vi "WT1800.vi"(7 "simulazione":bool, 8 "error in (no error)":errorcluster, 11 "Queue Name":string="WT1800_Q") -> (0 "error out":errorcluster, 2 "Stopped":bool)   [LabVIEW 2019]
uses:
  TypeDef/MISURE WT.ctl
  TypeDef/DEVICE NAME.ctl
  <vilib>/Utility/file.llb/Read From Spreadsheet File (string).vi
  <instrlib>/Yokogawa WT1800 Series/Public/Data/Low Level/Fetch Measurement (Normal).vi
  Globals.vi
  <instrlib>/Yokogawa WT1800 Series/Yokogawa WT1800 Series.lvlib
panel:
  out "Measurement":dbl[](array[numeric])
  in  "Number of Item (15)":i32=90 min=1 max=255
  in  "WT1800 Config ing":T1={"Wiring A (0: 1P2W)"=0, "Wiring B (0: 1P2W)"=0, "Wiring C (0: 1P2W)"=0, "V Range (12: 1000)"=12, "V Element (0: All)"=0, "A Element (0: All)"=0, "A Range (9: 5A)"=9, "A Sensor Ratio(mV/A) (10.0000) "=10.0, "Zero Cross Filter (0: OFF)"=0, "Line Filter (0: OFF)"=0, "PT Ratio (1.0000)"=1.0, "Scaling (F: OFF)"=FALSE, "CT Ratio (1.0000)"=1.0, "Scaling Factor (1.0000)"=1.0, "Filter Element (0: All)"=0, "Display Format (0: Numeric)"=0, "Normal Item Amount (1: 4)"=1, "Harmonics Item Amount (1: 4)"=1, "Average Type (0: OFF)"=0, "Average Count (2: 8)"=2, "A Range (9: 5A) 2"=9, "A Sensor Ratio(mV/A) (10.0000)  2"=10.0, "Zero Cross Filter (0: OFF) 2"=0, "Line Filter (0: OFF) 2"=0, "PT Ratio (1.0000) 2"=1.0, "Scaling (F: OFF) 2"=FALSE, "CT Ratio (1.0000) 2"=1.0, "Scaling Factor (1.0000) 2"=1.0, "CUT OFF FREQ"=0.0} {"Scaling Factor (1.0000) 2" min=0.0001 max=99999.9999 step=0.0001 format="%.4f"; "CT Ratio (1.0000) 2" min=0.0001 max=99999.9999 step=0.0001 format="%.4f"; "PT Ratio (1.0000) 2" min=0.0001 max=99999.9999 step=0.0001 format="%.4f"; "Line Filter (0: OFF) 2" items=["OFF", "500Hz", "5.5kHz"]; "Zero Cross Filter (0: OFF) 2" items=["OFF", "500Hz"]; "A Sensor Ratio(mV/A) (10.0000)  2" min=0.0001 max=99999.9999 step=0.0001 format="%.4f"; "A Range (9: 5A) 2" items=["AUTO", "10 mA", "20 mA", "50 mA", "100 mA", "200 mA", "500 mA", "1 A", "2 A", "5 A", "10 A", "20 A", "50 A", "S-AUTO", "50 mV", "100 mV", "250 mV", "500 mV", "1 V", "2.5 V", "5 V", "10 V"]; "Average Count (2: 8)" items=["2", "4", "8", "16", "32", "64", "128", "256"]; "Average Type (0: OFF)" items=["OFF", "Linear", "Exponent"]; "Harmonics Item Amount (1: 4)" items=["-", "4", "8", "16", "Single List", "Dual List", "Sigma List"]; "Normal Item Amount (1: 4)" items=["ALL", "4", "8", "16", "42", "78"]; "Display Format (0: Numeric)" items=["Numeric", "Wave", "Bar", "Vector", "Trend", "Numeric & Wave", "Numeric & Bar", "Numeric & Trend", "Wave & Bar", "Wave & Trend", "Bar & Trend", "Information"]; "Filter Element (0: All)" items=["All", "Element 1", "Element 2", "Element 3", "Element 4", "Element 5", "Element 6"]; "Scaling Factor (1.0000)" min=0.0001 max=99999.9999 step=0.0001 format="%.4f"; "CT Ratio (1.0000)" min=0.0001 max=99999.9999 step=0.0001 format="%.4f"; "PT Ratio (1.0000)" min=0.0001 max=99999.9999 step=0.0001 format="%.4f"; "Line Filter (0: OFF)" items=["OFF", "500Hz", "5.5kHz"]; "Zero Cross Filter (0: OFF)" items=["OFF", "500Hz"]; "A Sensor Ratio(mV/A) (10.0000)" min=0.0001 max=99999.9999 step=0.0001 format="%.4f"; "A Range (9: 5A)" items=["AUTO", "10 mA", "20 mA", "50 mA", "100 mA", "200 mA", "500 mA", "1 A", "2 A", "5 A", "10 A", "20 A", "50 A", "S-AUTO", "50 mV", "100 mV", "250 mV", "500 mV", "1 V", "2.5 V", "5 V", "10 V"]; "A Element (0: All)" items=["All", "Element 1", "Element 2", "Element 3", "Element 4", "Element 5", "Element 6"]; "V Element (0: All)" items=["All", "Element 1", "Element 2", "Element 3", "Element 4", "Element 5", "Element 6"]; "V Range (12: 1000)" items=["AUTO", "1.5", "3", "6", "10", "15", "30", "60", "100", "150", "300", "600", "1000"]; "Wiring C (0: 1P2W)" items=["1P2W", "1P3W", "3P3W", "3P4W", "3V3A", "NONE"]; "Wiring B (0: 1P2W)" items=["1P2W", "1P3W", "3P3W", "3P4W", "3V3A", "NONE"]; "Wiring A (0: 1P2W)" items=["1P2W", "1P3W", "3P3W", "3P4W", "3V3A"]}
  out "MISURE WT":T2
  out "VISA resource name":refnum<visa-resource-name>
  out "STATO":string
  out "LOOP TIME (ms)":u32
  # "ON\nOFF"
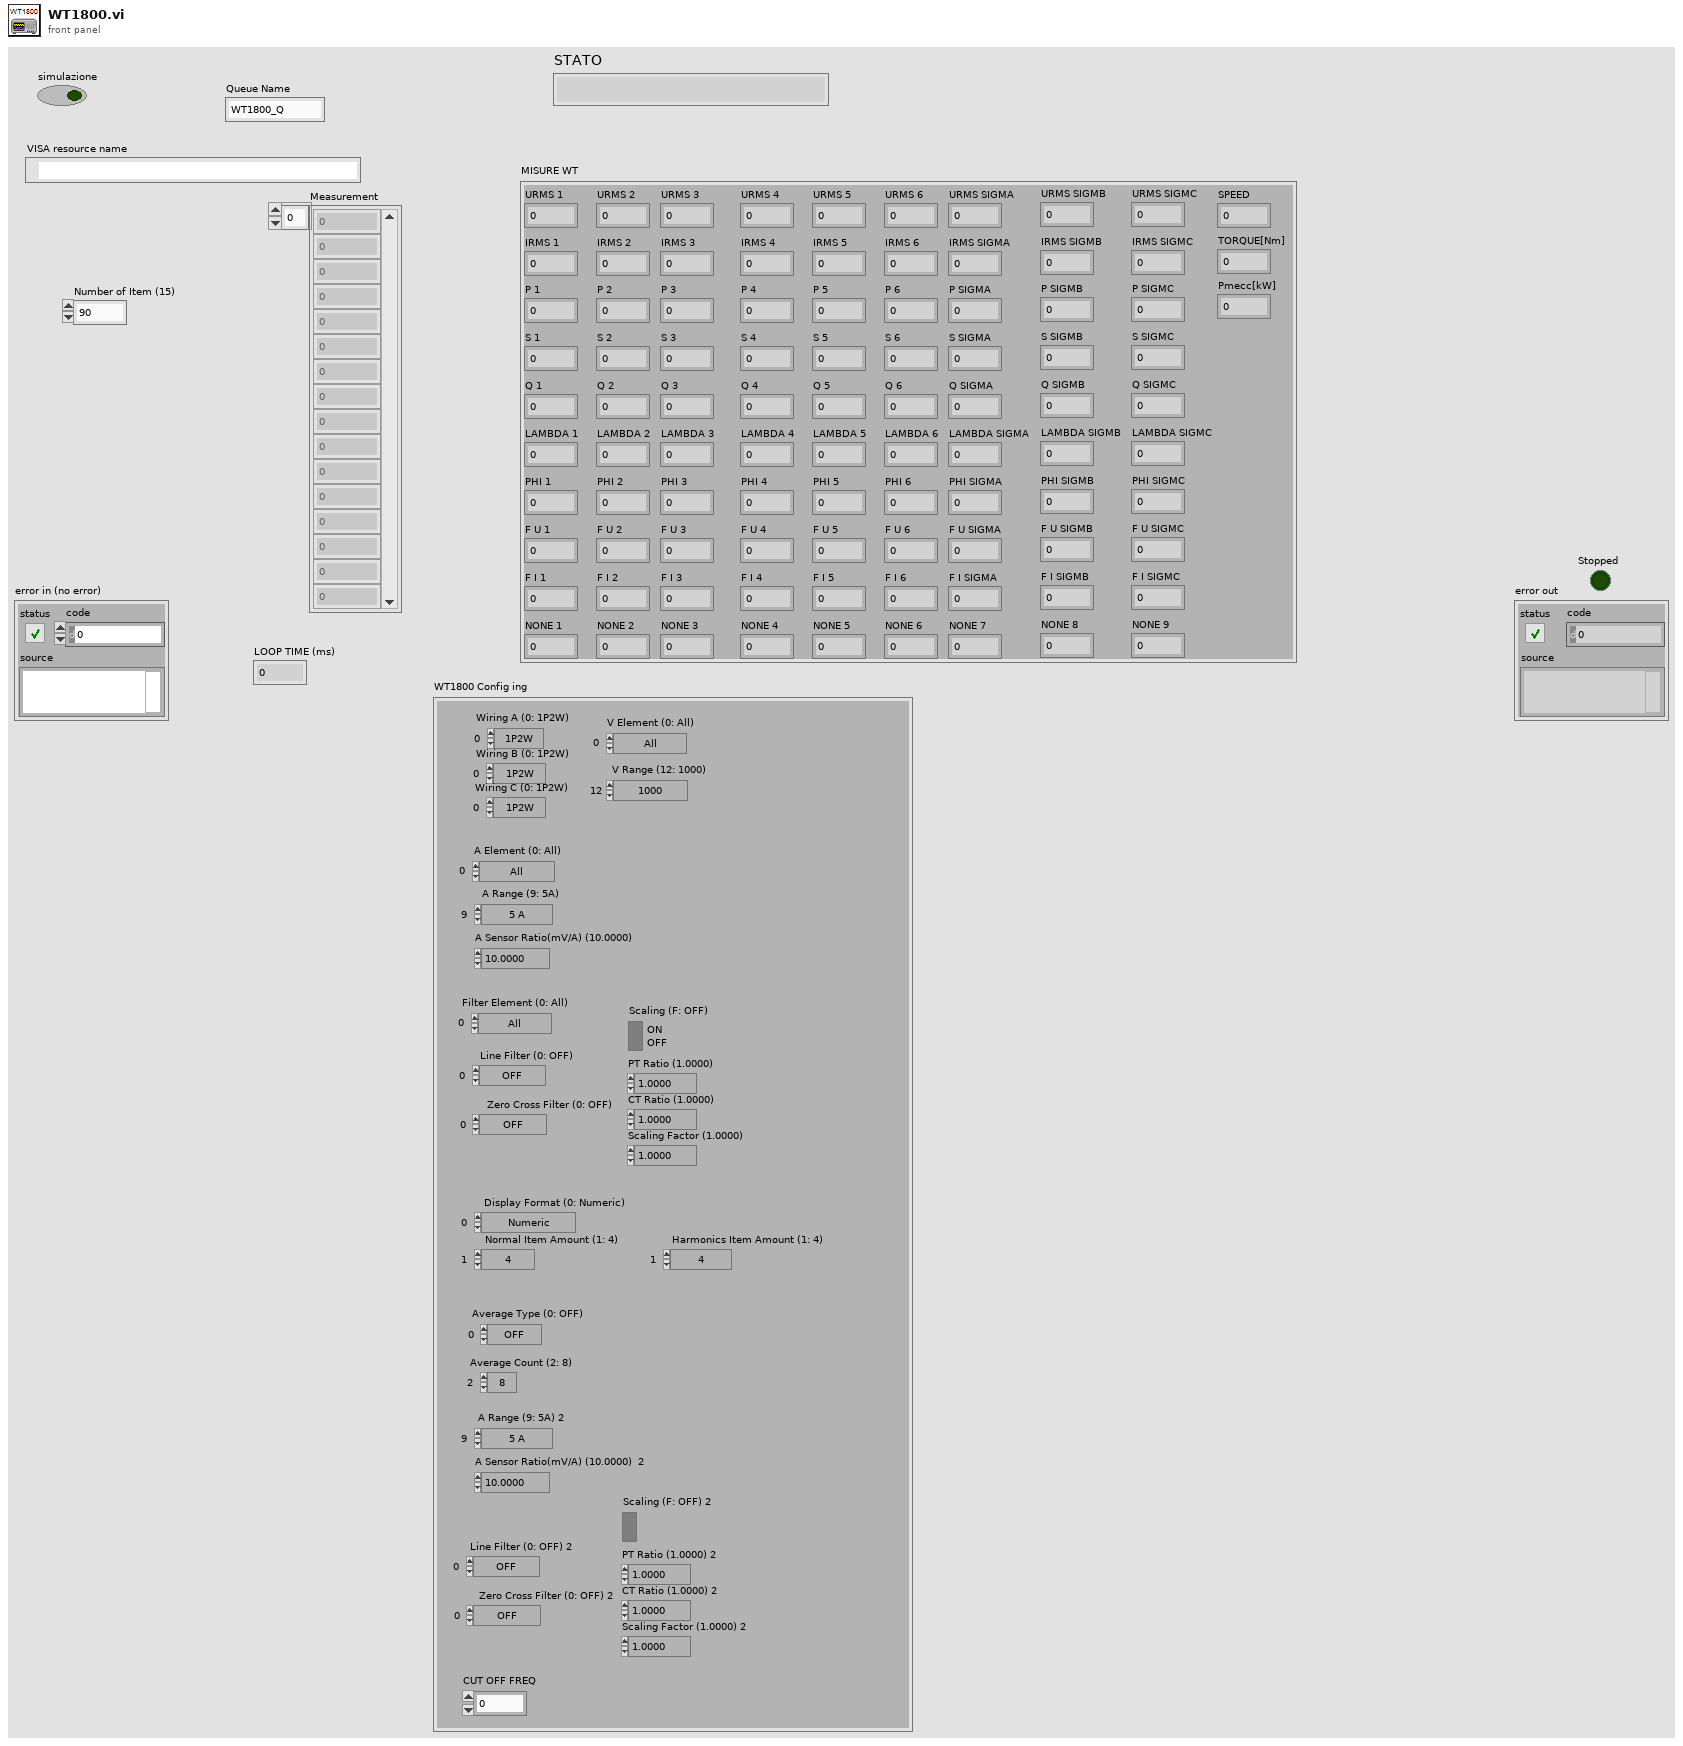
[diagram p1: front panel]
types:
  T1 = cluster{"Wiring A (0: 1P2W)":u16, "Wiring B (0: 1P2W)":u16, "Wiring C (0: 1P2W)":u16, "V Range (12: 1000)":u16, "V Element (0: All)":u16, "A Element (0: All)":u16, "A Range (9: 5A)":u16, "A Sensor Ratio(mV/A) (10.0000) ":dbl, "Zero Cross Filter (0: OFF)":u16, "Line Filter (0: OFF)":u16, "PT Ratio (1.0000)":dbl, "Scaling (F: OFF)":bool, "CT Ratio (1.0000)":dbl, "Scaling Factor (1.0000)":dbl, "Filter Element (0: All)":u16, "Display Format (0: Numeric)":u16, "Normal Item Amount (1: 4)":u16, "Harmonics Item Amount (1: 4)":u16, "Average Type (0: OFF)":u16, "Average Count (2: 8)":u16, "A Range (9: 5A) 2":u16, "A Sensor Ratio(mV/A) (10.0000)  2":dbl, "Zero Cross Filter (0: OFF) 2":u16, "Line Filter (0: OFF) 2":u16, "PT Ratio (1.0000) 2":dbl, "Scaling (F: OFF) 2":bool, "CT Ratio (1.0000) 2":dbl, "Scaling Factor (1.0000) 2":dbl, "CUT OFF FREQ":dbl}
  T2 = typedef "MISURE WT.ctl" = cluster{"URMS 1":dbl, "IRMS 1":dbl, "P 1":dbl, "S 1":dbl, "Q 1":dbl, "LAMBDA 1":dbl, "PHI 1":dbl, "F U 1":dbl, "F I 1":dbl, "NONE 1":dbl, "URMS 2":dbl, "IRMS 2":dbl, "P 2":dbl, "S 2":dbl, "Q 2":dbl, "LAMBDA 2":dbl, "PHI 2":dbl, "F U 2":dbl, "F I 2":dbl, "NONE 2":dbl, "URMS 3":dbl, "IRMS 3":dbl, "P 3":dbl, "S 3":dbl, "Q 3":dbl, "LAMBDA 3":dbl, "PHI 3":dbl, "F U 3":dbl, "F I 3":dbl, "NONE 3":dbl, "URMS 4":dbl, "IRMS 4":dbl, "P 4":dbl, "S 4":dbl, "Q 4":dbl, "LAMBDA 4":dbl, "PHI 4":dbl, "F U 4":dbl, "F I 4":dbl, "NONE 4":dbl, "URMS 5":dbl, "IRMS 5":dbl, "P 5":dbl, "S 5":dbl, "Q 5":dbl, "LAMBDA 5":dbl, "PHI 5":dbl, "F U 5":dbl, "F I 5":dbl, "NONE 5":dbl, "URMS 6":dbl, "IRMS 6":dbl, "P 6":dbl, "S 6":dbl, "Q 6":dbl, "LAMBDA 6":dbl, "PHI 6":dbl, "F U 6":dbl, "F I 6":dbl, "NONE 6":dbl, "URMS SIGMA":dbl, "IRMS SIGMA":dbl, "P SIGMA":dbl, "S SIGMA":dbl, "Q SIGMA":dbl, "LAMBDA SIGMA":dbl, "PHI SIGMA":dbl, "F U SIGMA":dbl, "F I SIGMA":dbl, "NONE 7":dbl, "URMS SIGMB":dbl, "IRMS SIGMB":dbl, "P SIGMB":dbl, "S SIGMB":dbl, "Q SIGMB":dbl, "LAMBDA SIGMB":dbl, "PHI SIGMB":dbl, "F U SIGMB":dbl, "F I SIGMB":dbl, "NONE 8":dbl, "URMS SIGMC":dbl, "IRMS SIGMC":dbl, "P SIGMC":dbl, "S SIGMC":dbl, "Q SIGMC":dbl, "LAMBDA SIGMC":dbl, "PHI SIGMC":dbl, "F U SIGMC":dbl, "F I SIGMC":dbl, "NONE 9":dbl, "SPEED":dbl, "TORQUE[Nm]":dbl, "Pmecc[kW]":dbl}
  T3 = typedef "DEVICE NAME.ctl" = enum16{"WATTMETRO", "APLUS", "PLC BANCO 1", "PLC RACK", "PLC BANCO 2", "PS", "NI cDAQ", "RESISTOMAT"}
  T4 = cluster{"Array of elements":cluster{"String":string, "variant":variant}[], "Single element":cluster{"String":string, "variant":variant}, "enque at\nopposite end (F)":bool, "no replications (F)":bool}
  T5 = cluster{"Measurement[0]":dbl, "Measurement[1]":dbl, "Measurement[2]":dbl, "Measurement[3]":dbl, "Measurement[4]":dbl, "Measurement[5]":dbl, "Measurement[6]":dbl, "Measurement[7]":dbl, "Measurement[8]":dbl, "Measurement[9]":dbl, "Measurement[10]":dbl, "Measurement[11]":dbl, "Measurement[12]":dbl, "Measurement[13]":dbl, "Measurement[14]":dbl, "Measurement[15]":dbl, "Measurement[16]":dbl, "Measurement[17]":dbl, "Measurement[18]":dbl, "Measurement[19]":dbl, "Measurement[20]":dbl, "Measurement[21]":dbl, "Measurement[22]":dbl, "Measurement[23]":dbl, "Measurement[24]":dbl, "Measurement[25]":dbl, "Measurement[26]":dbl, "Measurement[27]":dbl, "Measurement[28]":dbl, "Measurement[29]":dbl, "Measurement[30]":dbl, "Measurement[31]":dbl, "Measurement[32]":dbl, "Measurement[33]":dbl, "Measurement[34]":dbl, "Measurement[35]":dbl, "Measurement[36]":dbl, "Measurement[37]":dbl, "Measurement[38]":dbl, "Measurement[39]":dbl, "Measurement[40]":dbl, "Measurement[41]":dbl, "Measurement[42]":dbl, "Measurement[43]":dbl, "Measurement[44]":dbl, "Measurement[45]":dbl, "Measurement[46]":dbl, "Measurement[47]":dbl, "Measurement[48]":dbl, "Measurement[49]":dbl, "Measurement[50]":dbl, "Measurement[51]":dbl, "Measurement[52]":dbl, "Measurement[53]":dbl, "Measurement[54]":dbl, "Measurement[55]":dbl, "Measurement[56]":dbl, "Measurement[57]":dbl, "Measurement[58]":dbl, "Measurement[59]":dbl, "Measurement[60]":dbl, "Measurement[61]":dbl, "Measurement[62]":dbl, "Measurement[63]":dbl, "Measurement[64]":dbl, "Measurement[65]":dbl, "Measurement[66]":dbl, "Measurement[67]":dbl, "Measurement[68]":dbl, "Measurement[69]":dbl, "Measurement[70]":dbl, "Measurement[71]":dbl, "Measurement[72]":dbl, "Measurement[73]":dbl, "Measurement[74]":dbl, "Measurement[75]":dbl, "Measurement[76]":dbl, "Measurement[77]":dbl, "Measurement[78]":dbl, "Measurement[79]":dbl, "Measurement[80]":dbl, "Measurement[81]":dbl, "Measurement[82]":dbl, "Measurement[83]":dbl, "Measurement[84]":dbl, "Measurement[85]":dbl, "Measurement[86]":dbl, "Measurement[87]":dbl, "Measurement[88]":dbl, "Measurement[89]":dbl, "Measurement[90]":dbl, "Measurement[91]":dbl, "Measurement[92]":dbl}
  T6 = enum32{"Invalid", "Standard", "Closed", "Hidden", "Minimized", "Maximized"}
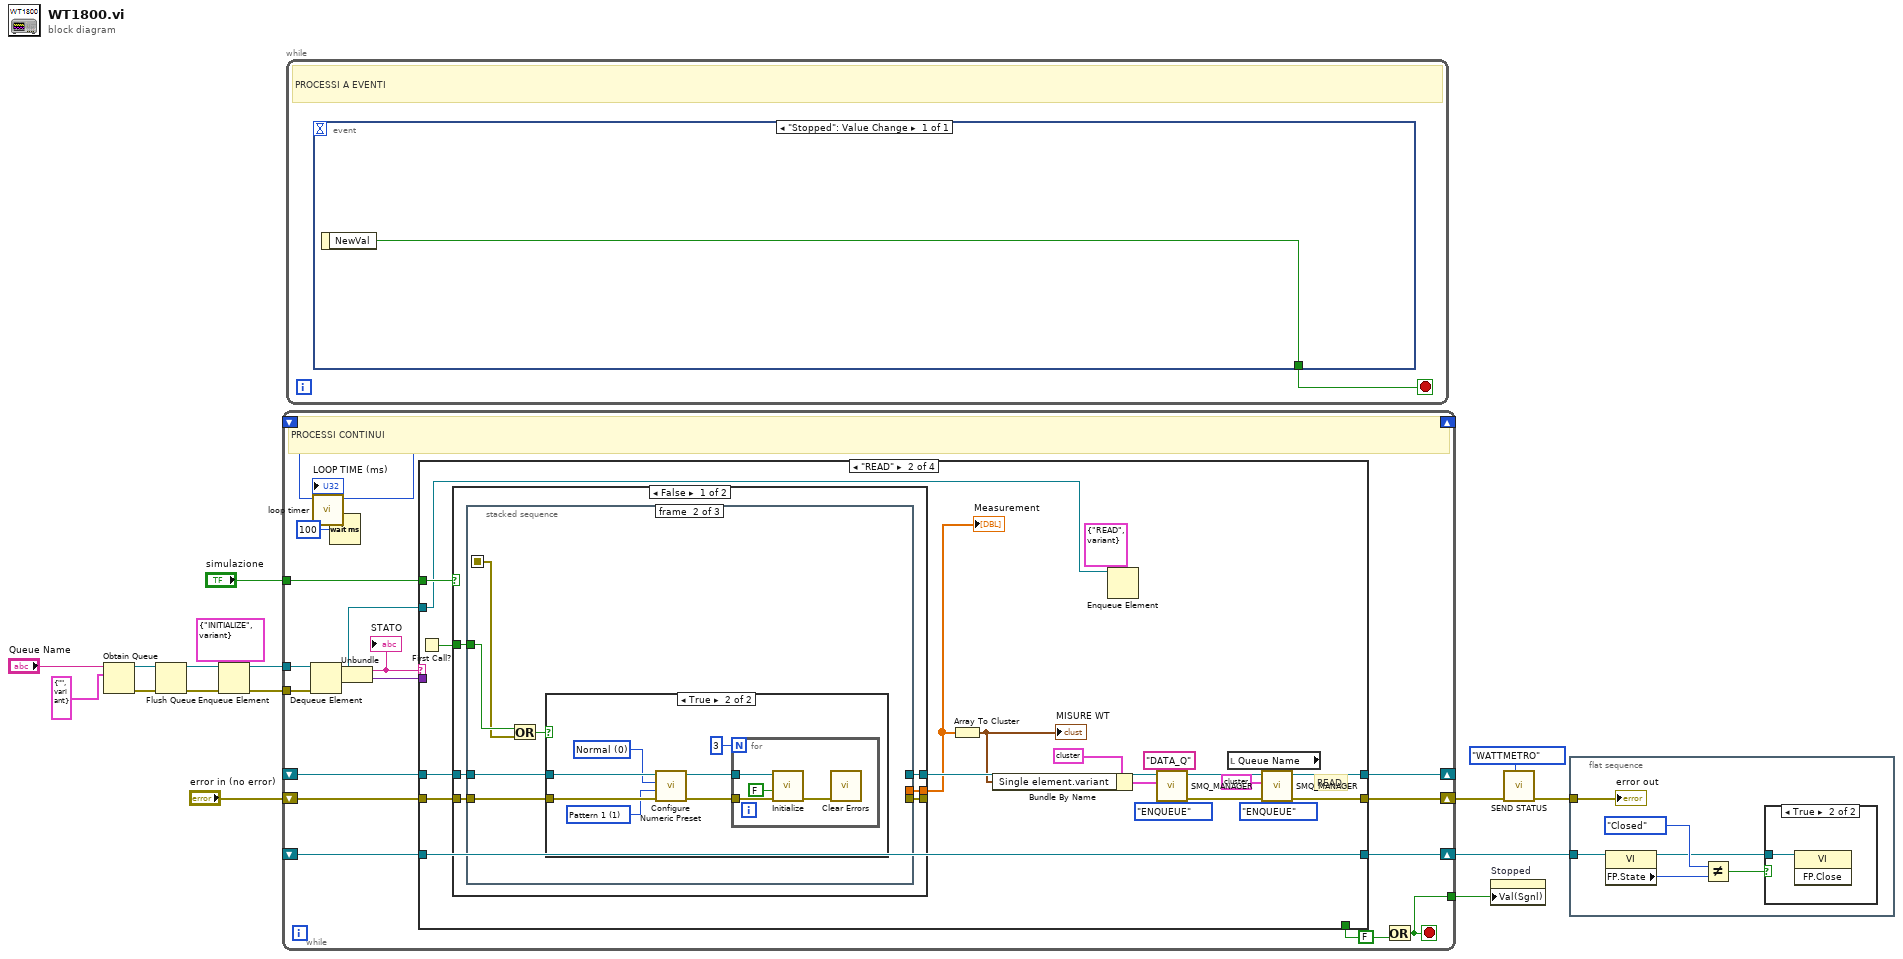
[diagram p0: block diagram]
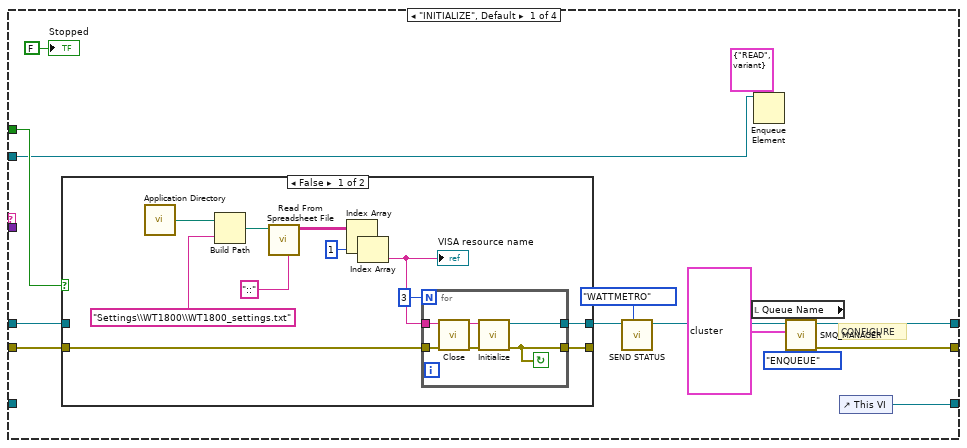
[diagram p3: hidden frame]
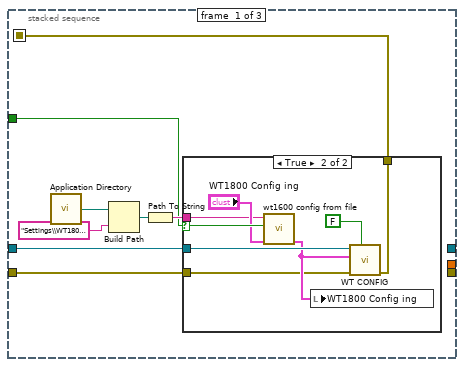
[diagram p5: hidden frame]
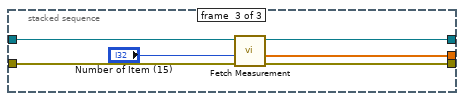
[diagram p8: hidden frame]
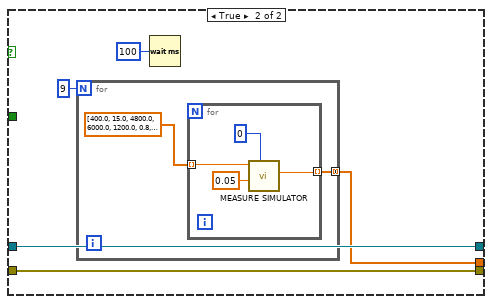
[diagram p9: hidden frame]
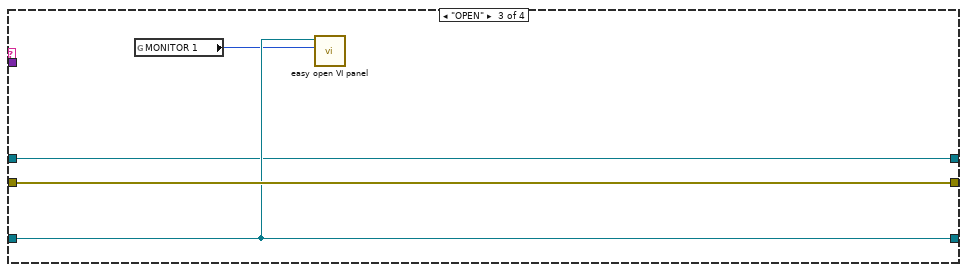
[diagram p10: hidden frame]
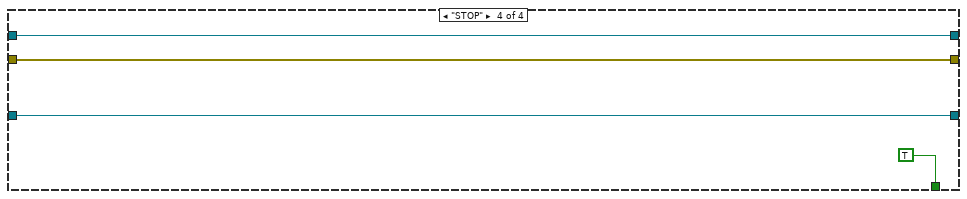
[diagram p11: hidden frame]
diagram:
  n1 = Obtain Queue(name (unnamed)="Queue Name", element data type=cluster{"String":string, "variant":variant} {"String"="", "variant"=variant} ("element")) -> (queue out=w5:refnum<queue>, error out=w4:errorcluster)  [unwired: 3 in, 1 out]
  n2 = Flush Queue(queue=w5, error in (no error)=w4) -> (queue out=w3:refnum<queue>, error out=w2:errorcluster)  [unwired: 1 out]
  n3 = Enqueue Element(queue=w3, element=cluster{"String":string, "variant":variant} {"String"="INITIALIZE", "variant"=variant}, error in (no error)=w2) -> (queue out=w12:refnum<queue>, error out=w11:errorcluster)  [unwired: 1 in, 1 out]
  n4 = while {
    shift-right: [w36] -> _
    shift-left: _ -> [w35]
    shift-right: [w33] -> w10
    shift-left: _ -> [w32]
    shift-right: [w29] -> w8
    shift-left: "error in (no error)" -> [w31]
    tunnel: w12 -> [w27]
    tunnel: w11 -> [w28]
    tunnel: [w23] -> w13
    tunnel: "simulazione" -> [w22]
    shift-right: [w20] -> _
    shift-left: _ -> [w19]
    stop <- w23 stop-if-true
    # "PROCESSI CONTINUI"
    n5 = Dequeue Element(queue=w27, error in (no error)=w28) -> (queue out=w17:refnum<queue>, element=w26:cluster{"String":string, "variant":variant})  [unwired: 1 in, 2 out]
    n6 = call <userlib>:"loop timer.vi"("millisecond timer IN"=w35) -> ("millisecond timer OUT"=w36:u32, "LOOP TIME (ms)"=→"LOOP TIME (ms)":u32)  [unwired: 9 in]
    n7 = Wait (ms)(milliseconds to wait=u32 100) -> ()  [unwired: 1 out]
    n8 = Unbundle(w26) -> ("String"=w25:string, "variant"=w24:variant)
    "STATO" <- w25
    n9 = case shown="\"READ\"" w25 {
      tunnel: [_ _ _ TRUE] -> w30
      tunnel: [w49 w87 w145 w149] -> w33
      tunnel: w32 -> [_ w87 w145 w149]
      tunnel: w31 -> [w47 w77 w146 w148]
      tunnel: [w43 w80 w146 w148] -> w29
      tunnel: w24 -> [_ _ _ _]
      tunnel: w22 -> [w41 w74 _ _]
      tunnel: [w42 w75 w143 w147] -> w20
      tunnel: w19 -> [w40 w76 w143 w147]
      tunnel: w17 -> [w38 w70 _ _]
      frame "INITIALIZE", Default {
        # "CONFIGURE"
        n10 = case shown="False" w41 {
          tunnel: w47 -> [w51 w68]
          tunnel: [w52 w68] -> _
          tunnel: [w53 w67] -> w42
          tunnel: w40 -> [_ w67]
          frame False {
            n11 = call <vilib>:"Application Directory.vi"() -> ("Application Directory"=w61:path)
            n12 = Build Path(base path=w61, name or relative path="Settings\\WT1800\\WT1800_settings.txt") -> (appended path=w59:path)
            n13 = call-poly <vilib>:"Read From Spreadsheet File.vi"("delimiter (\\t)"="::" ("delimiter (\\t)"), "file path (dialog if empty)"=w59) -> ("all rows"=w57:string[][])  [unwired: 5 in, 4 out]
            n14 = Index Array(array=w57, index (col)=1 ("disabled index (col)")) -> (element=w55:string[])  [unwired: 1 in]
            n15 = Index Array(array=w55) -> (element=w54:string)  [unwired: 1 in]
            "VISA resource name" <- w54
            n16 = for {
              N: 3 -> [_]
              tunnel: w54 -> [w62]
              tunnel: [w66] -> w53
              tunnel: [w65] -> w52
              tunnel: w51 -> [w64]
              stop <- w65 continue-if-true
              n17 = call <instrlib>:"Close.vi"("error in (no error)"=w64, "VISA resource name"=w62) -> ("error out"=w63:errorcluster)  [unwired: 9 in]
              n18 = call <instrlib>:"Initialize.vi"("error in (no error)"=w63, "VISA resource name"=w62) -> ("error out"=w65:errorcluster, "VISA resource name out"=w66:refnum<visa-resource-name>)  [unwired: 8 in]
            }
          }
          frame True {
          }
        }
        n19 = call "SEND STATUS.vi"("ELEMENT"=DEVICE_NAME."WATTMETRO") -> ()  [unwired: 10 in, 1 out]
        n20 = local read "Queue Name"() -> (w45:string)
        n21 = Enqueue Element(queue=w38, element=cluster{"String":string, "variant":variant} {"String"="READ", "variant"=variant}) -> ()  [unwired: 2 in, 3 out]
        n22 = call <userlib>:"SMQ_MANAGER.vi"("Function"=enum16{"INITIALIZE", "ENQUEUE", "STOP ALL"}."ENQUEUE", "Queue name"=w45, "Enqueue cluster"=T4 {"Array of elements"=[], "Single element"={"String"="READ", "variant"=variant}, "enque at\nopposite end (F)"=FALSE, "no replications (F)"=FALSE}) -> ("error out"=w43:errorcluster)  [unwired: 8 in]
        n23 = control-ref of="This VI"() -> (w49:refnum<vi>)
        "Stopped" <- FALSE ("Stop")
      }
      frame "READ" {
        # "READ"
        n24 = First Call?() -> (First Call?: T/F=w72:bool)
        n25 = case shown="False" w74 {
          tunnel: w77 -> [w89 w136]
          tunnel: [w92 w136] -> _
          tunnel: w76 -> [w90 w135]
          tunnel: [w93 w135] -> w75
          tunnel: [w88 w132] -> w73
          tunnel: w72 -> [w91 _]
          frame False {
            n26 = stacked-sequence {
              seq-local: [w94 _ _] -> [_ w111 _]
              tunnel: [_ _ w128] -> w93
              tunnel: [_ _ w129] -> w92
              tunnel: w91 -> [w97 w112 _]
              tunnel: w90 -> [w96 w113 w131]
              tunnel: w89 -> [w95 w114 w130]
              tunnel: [_ _ w127] -> w88
              frame #0 {
                n27 = call <vilib>:"Application Directory.vi"() -> ("Application Directory"=w99:path)
                n28 = Build Path(base path=w99, name or relative path="Settings\\WT1800\\WT1800_config.txt") -> (appended path=w100:path)
                n29 = Path To String(path=w100) -> (string=w101:string)
                n30 = case shown="True" w97 {
                  selector: w97 -> [_ w109]
                  tunnel: w96 -> [_ w107]
                  tunnel: w95 -> [_ w104]
                  tunnel: w101 -> [_ w103]
                  tunnel: [_ w102] -> w94
                  frame False {
                  }
                  frame True {
                    n31 = call "wt1600 config from file.vi"("WT1600 Config ing"="WT1800 Config ing", "leggi"=w109, "Path"=w103) -> ("output cluster"=w105:T1)  [unwired: 8 in]
                    n32 = local write "WT1800 Config ing"(w105) -> ()
                    n33 = call "WT CONFIG.vi"("WT 1600?"=FALSE, "error in (no error)"=w104, "WT1600 Config ing 2"=w105, "VISA Refnum in"=w107) -> ("error OUT"=w102:errorcluster)  [unwired: 6 in, 1 out]
                  }
                }
              }
              frame #1 {
                n34 = Or(x=w112, y=w111) -> (x .or. y?=w110:bool)
                n35 = case shown="True" w110 {
                  tunnel: w114 -> [_ w119]
                  tunnel: w113 -> [_ w120]
                  frame False {
                  }
                  frame True {
                    w115 = 1 items=["Pattern 1"=1, "Pattern 2"=2, "Pattern 3"=3, "Pattern 4"=4] ("Preset (Pattern 1)")
                    w116 = 0 items=["Normal", "Harmonics"] ("Target Item (0: Normal)")
                    n36 = call <instrlib>:"Configure Numeric Preset.vi"("error in (no error)"=w119, "Preset (Pattern 1)"=w115, "Target Item (0: Normal)"=w116, "VISA resource name"=w120) -> ("error out"=w117:errorcluster, "VISA resource name out"=w118:refnum<visa-resource-name>)  [unwired: 6 in]
                    n37 = for {
                      N: 3 -> [_]
                      tunnel: w117 -> [w125]
                      tunnel: w118 -> [w124]
                      n38 = call <instrlib>:"Initialize.vi"("error in (no error)"=w125, "Reset (True)"=FALSE, "VISA resource name"=w124) -> ("error out"=w122:errorcluster)  [unwired: 7 in, 1 out]
                      n39 = call <vilib>:"Clear Errors.vi"("error in (no error)"=w122) -> ()  [unwired: 5 in, 2 out]
                    }
                  }
                }
              }
              frame #2 {
                n40 = call-poly <instrlib>:"Fetch Measurement.vi"("error in (no error)"=w130, "Number of Item (15)"="Number of Item (15)", "VISA resource name"=w131) -> ("error out"=w129:errorcluster, "Measurement"=w127:dbl[], "VISA resource name out"=w128:refnum<visa-resource-name>)  [unwired: 6 in]
              }
            }
          }
          frame True {
            n41 = for {
              N: 9 -> [_]
              tunnel: [w137] -> w132 mode=concatenating
              n42 = for {
                tunnel: dbl[] [400.0, 15.0, 4800.0, 6000.0, 1200.0, 0.8, 0.0, 50.0, 50.0, nan] -> [w141] mode=indexing
                tunnel: [w139] -> w137 mode=indexing
                n43 = call <userlib>:"MEASURE SIMULATOR.vi"("delay (100)"=u32 0, "precision %"=0.05, "amplitude"=w141) -> ("value"=w139:dbl)  [unwired: 8 in]
              }
            }
            n44 = Wait (ms)(milliseconds to wait=u32 100) -> ()  [unwired: 1 out]
          }
        }
        "Measurement" <- w73
        n45 = Array To Cluster(array=w73) -> (cluster=w69:T5)
        "MISURE WT" <- w69
        n46 = Bundle By Name(cluster=T4 {"Array of elements"=[], "Single element"={"String"="READ WT", "variant"=variant}, "enque at\nopposite end (F)"=FALSE, "no replications (F)"=FALSE} ("Enqueue cluster"), "Single element.variant"=w69) -> (w83:T4)
        n47 = Enqueue Element(queue=w70, element=cluster{"String":string, "variant":variant} {"String"="READ", "variant"=variant}) -> ()  [unwired: 2 in, 3 out]
        n48 = call <userlib>:"SMQ_MANAGER.vi"("Function"=enum16{"INITIALIZE", "ENQUEUE", "STOP ALL"}."ENQUEUE", "Queue name"="DATA_Q", "Enqueue cluster"=w83) -> ("error out"=w81:errorcluster)  [unwired: 8 in]
        n49 = local read "Queue Name"() -> (w79:string)
        n50 = call <userlib>:"SMQ_MANAGER.vi"("Function"=enum16{"INITIALIZE", "ENQUEUE", "STOP ALL"}."ENQUEUE", "Queue name"=w79, "error in (no error)"=w81, "Enqueue cluster"=T4 {"Array of elements"=[], "Single element"={"String"="READ", "variant"=variant}, "enque at\nopposite end (F)"=FALSE, "no replications (F)"=FALSE}) -> ("error out"=w80:errorcluster)  [unwired: 7 in]
      }
      frame "OPEN" {
        n51 = global read "Globals.vi" "MONITOR 1"() -> (w144:u8)
        n52 = call <userlib>:"easy open VI panel.vi"("Monitor(1)"=w144, "VI in"=w145) -> ()  [unwired: 9 in, 1 out]
      }
      frame "STOP" {
      }
    }
    n53 = Or(x=FALSE, y=w30) -> (x .or. y?=w23:bool)
  }
  n54 = while {
    stop <- w151 stop-if-true
    # "PROCESSI A EVENTI"
    n55 = event shown="[0] \"Stopped\": Value Change" {
      selector: _ -> [_]
      dyn-events: _ -> [_]
      timeout: _ -> [_]
      tunnel: [w152] -> w151
      event "Stopped": Value Change {
        n56 = event-data() -> ("NewVal"=w152:bool)  [unwired: 1 in]
      }
    }
  }
  n57 = property on="Stopped" class="Bool (strict)"("Val(Sgnl)"=w13) -> ()  [unwired: 2 in, 2 out]
  n58 = call "SEND STATUS.vi"("ELEMENT"=DEVICE_NAME."WATTMETRO", "error in (no error)"=w8) -> ("error out"=w7:errorcluster)  [unwired: 9 in]
  n59 = flat-sequence {
    tunnel: w10 -> [w158]
    tunnel: w7 -> [w153]
    frame #0 {
      n60 = property class="VI"(reference=w158) -> (reference out=w154:refnum<vi>, "FP.State"=w157:T6)  [unwired: 1 in, 1 out]
      n61 = Not Equal?(x=T6."Closed", y=w157) -> (x != y?=w155:bool)
      n62 = case shown="True" w155 {
        tunnel: w154 -> [_ w159]
        frame False {
        }
        frame True {
          n63 = invoke class="VI" method="FP.Close"(reference=w159) -> ()  [unwired: 2 in, 3 out]
        }
      }
      "error out" <- w153
    }
  }
